vi "FilterMemory.vi"(7 "Reset":bool, 8 "error in (no error)":errorcluster, 9 "StateQueuesIn":string[](array[string]), 10 "NextStates":T1[](array[typedef]), 11 "StateNameIn":string="--Inte trådat--") -> (0 "error out":errorcluster, 1 "StateQueuesOut":cluster{"StateQueuesOut":string[]}[](array[cluster]), 2 "NextStates":cluster{"NextStates":T1[]}[](array[cluster]), 3 "StatesOut":string[](array[string]))   [LabVIEW 2016, in "StateReverse.lvclass"]
uses:
  <resource>/Framework/Providers/Open_GDS/UML/StateReverse_class/StateReverse.lvclass
  <resource>/Framework/Providers/Open_GDS/UML/StateReverse_class/NextStateAction.ctl
  <resource>/Framework/Providers/Open_GDS/UML/StateReverse_class/StateAction.ctl
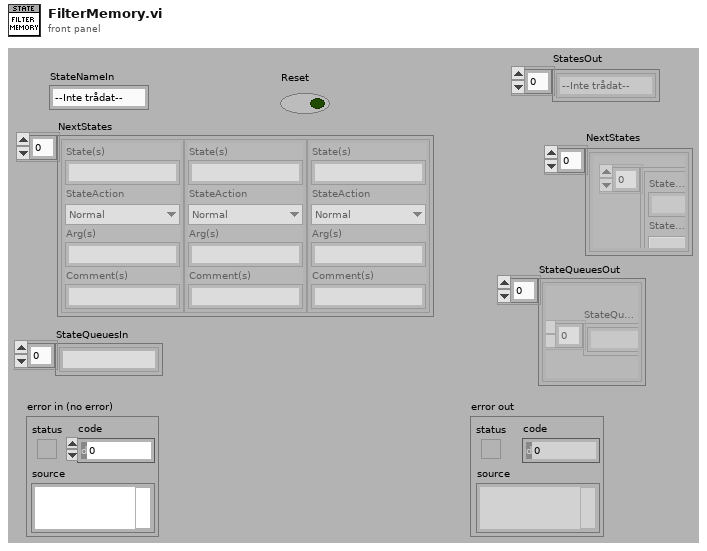
[diagram p1: front panel]
types:
  T1 = typedef "StateReverse.lvclass/NextStateAction.ctl" = cluster{"State(s)":string, "StateAction":T2, "Arg(s)":string, "Comment(s)":string}
  T2 = typedef "StateReverse.lvclass/StateAction.ctl" = enum16{"Normal", "AddInBeggining", "AddInEnd", "AddIfNothingInQueue"}
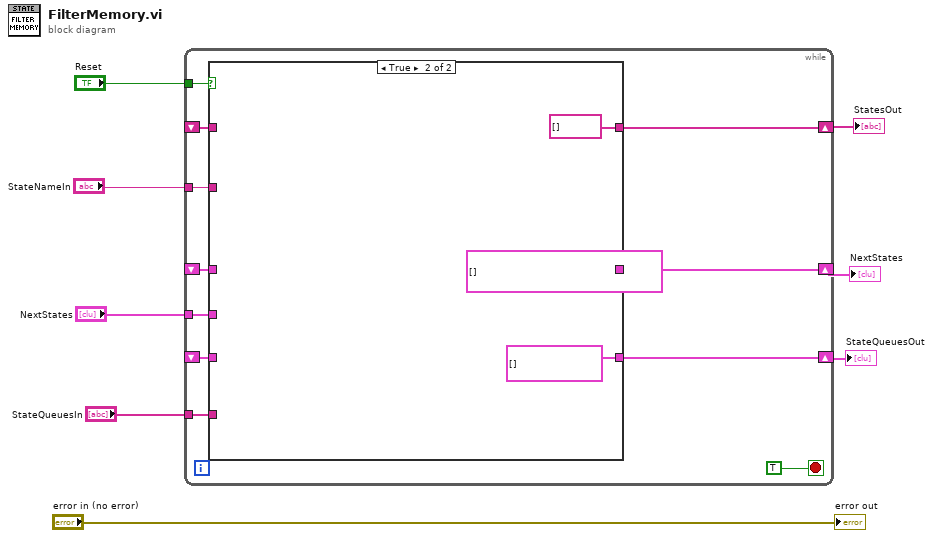
[diagram p0: block diagram]
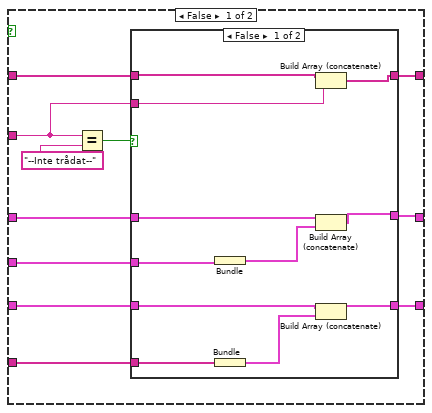
[diagram p2: hidden frame]
diagram:
  n1 = while {
    tunnel: "StateNameIn" -> [w19]
    tunnel: "Reset" -> [w18]
    shift-right: [w15] -> w4
    shift-left: _ -> [w16]
    shift-right: [w13] -> w5
    shift-left: _ -> [w14]
    shift-right: [w11] -> w3
    shift-left: _ -> [w12]
    tunnel: "NextStates" -> [w10]
    tunnel: "StateQueuesIn" -> [w9]
    stop <- TRUE stop-if-true
    n2 = case shown="True" w18 {
      tunnel: w19 -> [w22 _]
      tunnel: w16 -> [w28 _]
      tunnel: [w27 string[] [] ("StatesOut")] -> w15
      tunnel: w14 -> [w26 _]
      tunnel: [w25 cluster{"NextStates":T1[]}[] [] ("NextStates")] -> w13
      tunnel: w12 -> [w24 _]
      tunnel: [w23 cluster{"StateQueuesOut":string[]}[] [] ("StateQueuesOut")] -> w11
      tunnel: w10 -> [w21 _]
      tunnel: w9 -> [w20 _]
      frame False {
        n3 = Equal?(x=w22, y="--Inte trådat--" ("StateNameIn")) -> (x = y?=w29:bool)
        n4 = case shown="False" w29 {
          tunnel: w28 -> [w41 w44]
          tunnel: [w40 w44] -> w27
          tunnel: [w36 w43] -> w25
          tunnel: w26 -> [w38 w43]
          tunnel: [w35 w42] -> w23
          tunnel: w24 -> [w37 w42]
          tunnel: w22 -> [w39 _]
          tunnel: w21 -> [w32 _]
          tunnel: w20 -> [w34 _]
          frame False {
            n5 = Bundle("NextStates"=w32) -> (w31:cluster{"NextStates":T1[]})  [unwired: 1 in]
            n6 = Bundle("StateQueuesIn"=w34) -> (w33:cluster{"StateQueuesIn":string[]})  [unwired: 1 in]
            n7 = Build Array (concatenate)(w41, w39) -> (w40:string[])
            n8 = Build Array (concatenate)(w38, w31) -> (w36:cluster{"NextStates":T1[]}[])
            n9 = Build Array (concatenate)(w37, w33) -> (w35:cluster{"StateQueuesIn":string[]}[])
          }
          frame True {
          }
        }
      }
      frame True {
      }
    }
  }
  "StatesOut" <- w4
  "NextStates" <- w5
  "StateQueuesOut" <- w3
  "error out" <- "error in (no error)"
